vi "DLUOutputuffer.vi"(6 "Ready for Output":bool, 9 "Input Valid":bool, 10 "Input Data":T1) -> (1 "Output Valid":bool, 2 "Output Data":cluster{"Data to Node":u64, "Node Id":u16}, 4 "Ready For Input":bool)   [LabVIEW 2014, in "IO Node Logic Template.lvlib"]
uses:
  IO Node Logic Template.lvlib
  <vilib>/SPIAPI/Controls/SPI Response Information.ctl
  <vilib>/rvi/Emulation/niFpgaSctlEmulationGetInTimedLoop.vi
  <vilib>/rvi/DataTransferAndStorage/Container/Common/niFpgaContainerGetUniqueNameForEmu.vi
  <vilib>/rvi/DataTransferAndStorage/Container/Common/niFpgaContainerSetEmuInfo.vi
  <vilib>/rvi/eio/common/nirviEmuReportErrorAndStop.vi
  <vilib>/rvi/DataTransferAndStorage/Container/Common/niFpgaContainerExecOnDevCompGetState.vi
  <vilib>/rvi/Emulation/niFpgaEmulationIsFPGAContextNoSignature.vi
  <vilib>/rvi/errors/niFpgaSetErrorForExecOnDevCompSimple.vi
  <vilib>/rvi/FIFO/Fifo_Resource/nirvififoEmulationSetSize.vi
  <vilib>/rvi/FIFO/Fifo_Resource/nirviFifoEmulationQueueMgr.vi
  <instcachedir>/0/nirviFifoEmulationQueueMgr_E5CAEC123FF24DC58D834DCA3CDAA9B5.lvgen/nirviFifoEmulationQueueMgr_E5CAEC123FF24DC58D834DCA3CDAA9B5_006.vi
  <vilib>/rvi/FIFO/Fifo_Resource/nirvififoEmulationDetermineInputValidOut.vi
  <vilib>/rvi/FIFO/Fifo_Resource/nirvififoEmulationCreateLock.vi
  <vilib>/rvi/Emulation/niFpgaProcessEmulError.vi
  <vilib>/rvi/FIFO/Fifo_Resource/nirvififoEmulationObtainLock.vi
  <vilib>/rvi/FIFO/Fifo_Resource/nirvififoEmulationReleaseLock.vi
  <vilib>/rvi/occurrence/nirviWaitOnOccurrenceBase.vi
  <vilib>/rvi/errors/nirviReportUnexpectedCaseInternalError.vi
  <vilib>/rvi/errors/nirviReportUnexpectedCaseInternalError (U32).vi
  <vilib>/rvi/interface/RandomDataEmulation/niFpgaRandomDataHandleErrors.vi
  <vilib>/rvi/LocalResourceManager/LocalResourceManager.xnode
  <vilib>/rvi/DataTransferAndStorage/Container/XNode/niFpgaContainer.xnode
  <vilib>/rvi/FIFO/Fifo_Resource/niFpgaFifoEmulationRefIn.vi
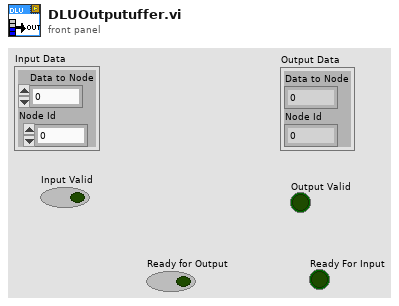
[diagram p1: front panel]
types:
  T1 = typedef "SPI Response Information.ctl" = cluster{"Data to Node":u64, "Node Id":u16}
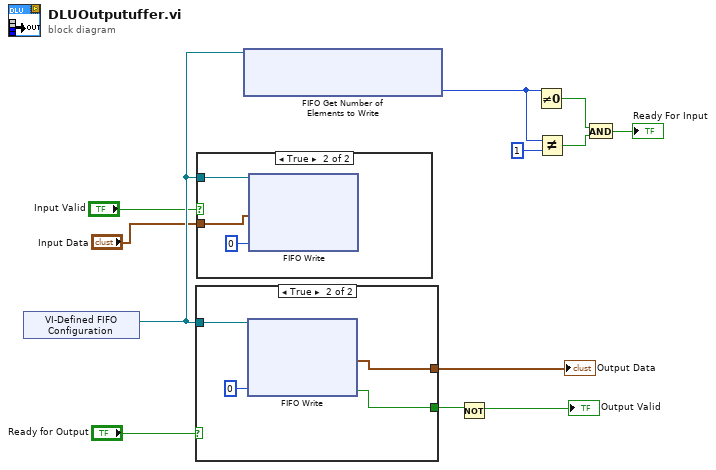
[diagram p0: block diagram]
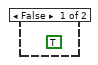
[diagram p2: hidden frame]
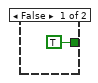
[diagram p3: hidden frame]
diagram:
  n1 = xnode "VI-Defined FIFO Configuration"() -> ("FIFO Out"=w12:refnum<k21>)
  n2 = case shown="True" "Ready for Output" {
    tunnel: w12 -> [_ w16]
    tunnel: [_ w15] -> w1
    tunnel: [TRUE ("Timed Out?") w14] -> w4
    frame False {
    }
    frame True {
      n3 = xnode "FIFO Write"("Timeout"=0, "FIFO In"=w16) -> ("Element"=w15:cluster{"Data to Node":u64, "Node Id":u16}, "Timed Out?"=w14:bool)  [unwired: 1 out]
    }
  }
  "Output Data" <- w1
  n4 = case shown="True" "Input Valid" {
    tunnel: w12 -> [_ w19]
    tunnel: "Input Data" -> [_ w18]
    frame False {
      (unwired) TRUE ("Timed Out?")
    }
    frame True {
      n5 = xnode "FIFO Write"("Element"=w18, "Timeout"=0, "FIFO In"=w19) -> ()  [unwired: 2 out]
    }
  }
  n6 = xnode "FIFO Get Number of Elements to Write"("FIFO In"=w12) -> ("Number of Elements to Write"=w11:u32)  [unwired: 1 out]
  n7 = Not(x=w4) -> (.not. x?=→"Output Valid":bool)
  n8 = Not Equal To 0?(x=w11) -> (x != 0?=w9:bool)
  n9 = Not Equal?(x=w11, y=u32 1) -> (x != y?=w10:bool)
  n10 = And(x=w9, y=w10) -> (x .and. y?=→"Ready For Input":bool)
